vi "open_climber.vi"(8 "error in (no error)":errorcluster) -> (0 "error out":errorcluster)   [LabVIEW 2020]
uses:
  <vilib>/Rock Robotics/WPI/ThirdParty/Phoenix-LabVIEW/Motor Controller/Controls/CTRE_Phoenix_MotorControl_NeutralMode.ctl
  Status Frame Stuff/Talon Status Config Array.ctl
  Status Frame Stuff/Talon Status Frame Setting.ctl
  <vilib>/Rock Robotics/WPI/ThirdParty/Phoenix-LabVIEW/Motor Controller/Controls/CTRE_Phoenix_MotorControl_StatusFrameEnhanced.ctl
  Status Frame Stuff/STATUS_Period.ctl
panel:
  in  "Climber PIDF":T1={"Set Constants"=TRUE, "P"=0.45, "I"=0.0, "D"=0.0, "F"=0.0, "I Zone"=0.0, "Cruise Velocity"=20000, "Acceleration"=40000, "Percent Deadband"=0.7}
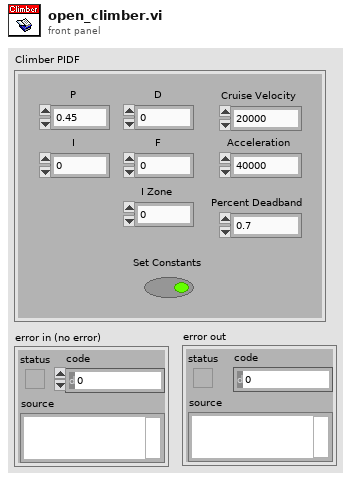
[diagram p1: front panel]
types:
  T1 = cluster{"Set Constants":bool, "P":dbl, "I":dbl, "D":dbl, "F":dbl, "I Zone":dbl, "Cruise Velocity":i32, "Acceleration":i32, "Percent Deadband":dbl}
  T2 = typedef "CTRE_Phoenix_MotorControl_NeutralMode.ctl" = enum8{"EEPROMSetting", "Override to Coast", "Override to Brake"}
  T3 = typedef "Talon Status Config Array.ctl" = T4[]
  T4 = typedef "Talon Status Frame Setting.ctl" = cluster{"Status Frame Enum":T5, "STATUS_Period":T6}
  T5 = typedef "CTRE_Phoenix_MotorControl_StatusFrameEnhanced.ctl" = u16
  T6 = typedef "STATUS_Period.ctl" = i32
  T7 = typedef "WPI_MotorControlDeviceRef.ctl" = cluster{"DeviceStatus":errorcluster, "Type":T8, "PWM":cluster{"PWM Channel":T9, "DeadBand":T10}, "CAN":cluster{"Device Number":u8, "SetOutput VI Ref":variant, "GetOutput VI Ref":variant, "Enable VI Ref":variant, "Disable VI Ref":variant, "Data":variant}, "Invert":bool, "DIO PWM":cluster{"PWM \"Enable\" Channel":T9, "DIOChannel":T11, "PWM Rate":dbl}}
  T8 = typedef "WPI_MotorControlType.ctl" = enum16{"PWM", "CAN", "DIO PWM"}
  T9 = typedef "FPGA_DIOPWMChannel.ctl" = enum8{"PWM 0", "PWM 1", "PWM 2", "PWM 3", "PWM 4", "PWM 5", "PWM 6", "PWM 7", "PWM 8", "PWM 9", "PWM MXP 0", "PWM MXP 1", "PWM MXP 2", "PWM MXP 3", "PWM MXP 4", "PWM MXP 5", "PWM MXP 6", "PWM MXP 7", "PWM MXP 8", "PWM MXP 9", "Invalid"}
  T10 = typedef "WPI_PWMDeadband.ctl" = cluster{"Name":string, "maxPositivePwm":i32, "minPositivePwm":i32, "centerPwm":i32, "maxNegativePwm":i32, "minNegativePwm":i32, "angularRange":u16}
  T11 = typedef "FPGA_DIOChannel.ctl" = enum8{"DIO 0", "DIO 1", "DIO 2", "DIO 3", "DIO 4", "DIO 5", "DIO 6", "DIO 7", "DIO 8", "DIO 9", "DIO MXP 0", "DIO MXP 1", "DIO MXP 2", "DIO MXP 3", "DIO MXP 4", "DIO MXP 5", "DIO MXP 6", "DIO MXP 7", "DIO MXP 8", "DIO MXP 9", "DIO MXP 10", "DIO MXP 11", "DIO MXP 12", "DIO MXP 13", "DIO MXP 14", "DIO MXP 15", "SPI Port CS1", "SPI Port CS2", "SPI Port CS3", "SPI Port MISO", "SPI Port MOSI", "Invalid"}
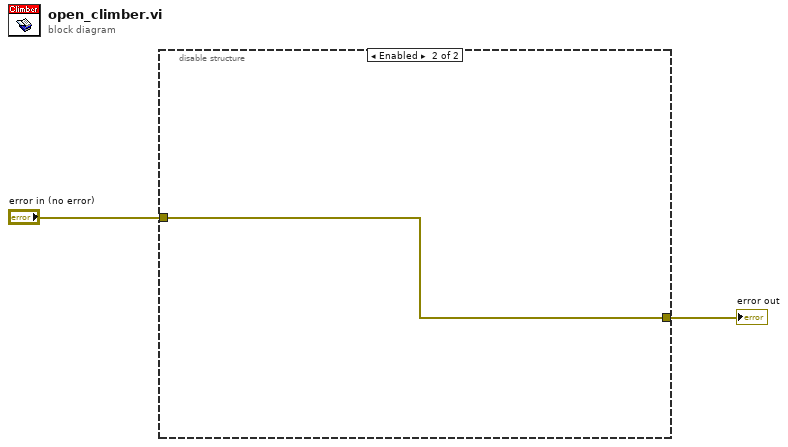
[diagram p0: block diagram]
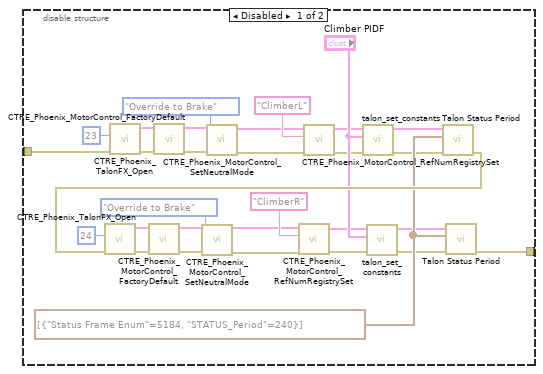
[diagram p2: hidden frame]
diagram:
  n1 = disable-structure shown="Enabled" {
    disable-tunnel: [w33 w34] -> w2
    disable-tunnel: "error in (no error)" -> [w32 w34]
    frame Disabled {
      w30 = T3 [{"Status Frame Enum"=5184, "STATUS_Period"=240}] ("Drive Status Config")
      n2 = call <vilib>:"CTRE_Phoenix_TalonFX_Open.vi"("error in"=w32, "Device Number"=u8 23) -> ("error out"=w16:errorcluster, "PhoenixMotorControlDevRef"=w17:T7)  [unwired: 8 in]
      n3 = call <vilib>:"CTRE_Phoenix_MotorControl_FactoryDefault.vi"("error in"=w16, "PhoenixMotorControlDevRef"=w17) -> ("error out"=w21:errorcluster, "PhoenixMotorControlDevRef"=w20:T7)  [unwired: 8 in]
      n4 = call <vilib>:"CTRE_Phoenix_MotorControl_SetNeutralMode.vi"("error in (no error)"=w21, "Motor Control Neutral Mode"=CTRE_Phoenix_MotorControl_NeutralMode."Override to Brake", "PhoenixMotorControlDevRef"=w20) -> ("error out"=w13:errorcluster, "PhoenixMotorControlDevRef"=w14:T7)  [unwired: 7 in]
      n5 = call <vilib>:"CTRE_Phoenix_MotorControl_RefNumRegistrySet.vi"("error in (no error)"=w13, "refnum name"="ClimberL", "PhoenixMotorControlDevRef"=w14) -> ("error out"=w11:errorcluster, "PhoenixMotorControlDevRef"=w12:T7)  [unwired: 7 in]
      n6 = call "talon_set_constants.vi"("error in"=w11, "Constants"="Climber PIDF", "PhoenixMotorControlDevRef"=w12) -> ("error out"=w4:errorcluster, "PhoenixMotorControlDevRef"=w3:T7)  [unwired: 7 in]
      n7 = call "Talon Status Period.vi"("error in (no error)"=w4, "Status Config Array"=w30, "PhoenixMotorControlDevRef"=w3) -> ("error out"=w31:errorcluster)  [unwired: 7 in, 1 out]
      n8 = call <vilib>:"CTRE_Phoenix_TalonFX_Open.vi"("error in"=w31, "Device Number"=u8 24) -> ("error out"=w23:errorcluster, "PhoenixMotorControlDevRef"=w24:T7)  [unwired: 8 in]
      n9 = call <vilib>:"CTRE_Phoenix_MotorControl_FactoryDefault.vi"("error in"=w23, "PhoenixMotorControlDevRef"=w24) -> ("error out"=w28:errorcluster, "PhoenixMotorControlDevRef"=w27:T7)  [unwired: 8 in]
      n10 = call <vilib>:"CTRE_Phoenix_MotorControl_SetNeutralMode.vi"("error in (no error)"=w28, "Motor Control Neutral Mode"=CTRE_Phoenix_MotorControl_NeutralMode."Override to Brake", "PhoenixMotorControlDevRef"=w27) -> ("error out"=w9:errorcluster, "PhoenixMotorControlDevRef"=w10:T7)  [unwired: 7 in]
      n11 = call <vilib>:"CTRE_Phoenix_MotorControl_RefNumRegistrySet.vi"("error in (no error)"=w9, "refnum name"="ClimberR", "PhoenixMotorControlDevRef"=w10) -> ("error out"=w8:errorcluster, "PhoenixMotorControlDevRef"=w7:T7)  [unwired: 7 in]
      n12 = call "talon_set_constants.vi"("error in"=w8, "Constants"="Climber PIDF", "PhoenixMotorControlDevRef"=w7) -> ("error out"=w6:errorcluster, "PhoenixMotorControlDevRef"=w5:T7)  [unwired: 7 in]
      n13 = call "Talon Status Period.vi"("error in (no error)"=w6, "Status Config Array"=w30, "PhoenixMotorControlDevRef"=w5) -> ("error out"=w33:errorcluster)  [unwired: 7 in, 1 out]
    }
    frame Enabled {
    }
  }
  "error out" <- w2
